vi "Dashboard Main.vi"() -> ()   [LabVIEW 2016]
uses:
  <vilib>/Utility/miscctls.llb/LVRowAndColumnTypeDef.ctl
  <vilib>/event_ctls.llb/eventvkey.ctl
  <vilib>/Rock Robotics/Network Tables/NT Read Numeric Array.vi
  <vilib>/Rock Robotics/Network Tables/NT Read Boolean.vi
  <vilib>/Rock Robotics/WPI/Dashboard/WPI_DashboardLogging Global.vi
panel:
  in  "Camera Settings Right":T1={"Frame Rate"=30, "Compression"=30, "Size"=1, "DB Camera Config"=FALSE} {"Frame Rate" scale=1.0..30.0; "Compression" scale=100.0..-1.0; "Size" items=["640x480", "320x240", "160x120"]}
  in  "Camera Name Right":string(combo)="No Camera Selection"
  out "Camera Info":cluster{"Mbps LED":bool, "Mbps":dbl, "fps":dbl} {"fps" format="%#.1g"; "Mbps" format="%#.1g"}
  in  "Camera Settings":T1={"Frame Rate"=30, "Compression"=30, "Size"=1, "DB Camera Config"=FALSE} {"Frame Rate" scale=1.0..30.0; "Compression" scale=100.0..-1.0; "Size" items=["640x480", "320x240", "160x120"]}
  in  "TCP":refnum<k5>
  in  "Rec Mode":enum32{"Stop", "Record", "Playback"}(radio)
  out "Robot IP":string
  out "Image Message":string="Timeout in Camera Communications"
  in  "Dashboard Tab":T2(tab)
  out "Centered? Cyan is go":bool
  in  "Select Auto":string(combo)="Select Autonomous ..."
  out "NT Connection":bool
  out "MotorChart R":cluster{"Numeric":dbl, "Numeric":dbl}(graph)
  out "MotorChart L":cluster{"Numeric":dbl, "Numeric":dbl}(graph)
  out "MotorSliders R":cluster{"MotorSlide1":dbl, "MotorSlide2":dbl} {"MotorSlide2" scale=-1.0..1.0 scale format="%#_2e"; "MotorSlide1" scale=-1.0..1.0 scale format="%#_2e"}
  out "MotorSliders L":cluster{"MotorSlide1":dbl, "MotorSlide2":dbl} {"MotorSlide2" scale=-1.0..1.0 scale format="%#_2e"; "MotorSlide1" scale=-1.0..1.0 scale format="%#_2e"}
  out "Gyro":dbl(knob) scale=0.0..360.0
  out "JS1 Z":dbl(slide) scale=-1.0..1.0 scale format="%#_2e"
  out "JS1 Graph":cluster{"X":dbl, "Y":dbl}[](graph)
  out "JS1 Buttons":T3
  out "JS2 Z":dbl(slide) scale=-1.0..1.0 scale format="%#_2e"
  out "JS2 Graph":cluster{"X":dbl, "Y":dbl}[](graph)
  out "JS2 Buttons":T3
  out "Mode":T4(ring)=enum."Auto Disabled"
  out "Camera Image Right":T5(plugin-control)
  in  "DB/String 9":string
  in  "DB/String 8":string
  in  "DB/String 7":string
  in  "DB/String 6":string
  in  "DB/String 5":string
  in  "DB/String 4":string
  in  "DB/String 3":string
  in  "DB/String 2":string
  in  "DB/String 1":string
  in  "DB/String 0":string
  in  "DB/Slider 0":dbl(slide) scale=0.0..5.0
  in  "DB/Slider 1":dbl(slide) scale=0.0..5.0
  in  "DB/Slider 2":dbl(slide) scale=0.0..5.0
  in  "DB/Slider 3":dbl(slide) scale=0.0..5.0
  out "DB/LED 3":bool
  out "DB/LED 2":bool
  out "DB/LED 1":bool
  out "DB/LED 0":bool
  in  "DB/Button 3":bool
  in  "DB/Button 2":bool
  in  "DB/Button 1":bool
  in  "DB/Button 0":bool caption="New Name"
  in  "Test Slider":dbl(slide) scale=0.0..100.0 scale format="%#_3g"
  in  "On/Off":bool caption="Solenoid"
  in  "Test Name":u16(ring) items=["Select the test to run..."]
  in  "Test Tree":string(tree)
  in  "Motor":cluster{"Value":dbl, "Enable":bool} {"Value" scale=-1.0..1.0 scale format="%#_3g"}
  out "Progress":T6 {"Test Progress" scale=0.0..100.0}
  in  "Rev/Fwd":cluster{"Forward":bool, "Reverse":bool}
  in  "Test Ring":u16(ring) items=["Monochrome", "Color"]
  out "Cmd Status":string
  in  "Execute Command":bool
  in  "Command Params":string[][](table)
  in  "Command Selection":i32(listbox)
  in  "CheckList":i32(listbox)
  out "Tree":string(tree)
  out "Camera Image":T5(plugin-control)
  out "Background":bool
  in  "Camera Name":string(combo)="No Camera Selection"
  # "HW"
  # "HW"
  # "Joysticks"
  # "Drive Motors"
  # "Front"
  # "Right"
  # "Left"
  # "Back"
  # "This tab is a great place for autonomous settings and robot-specific values.\nPlace controls and indicators inside this tab and match name to\nDashboard Variables on robot. You can also delete this comment."
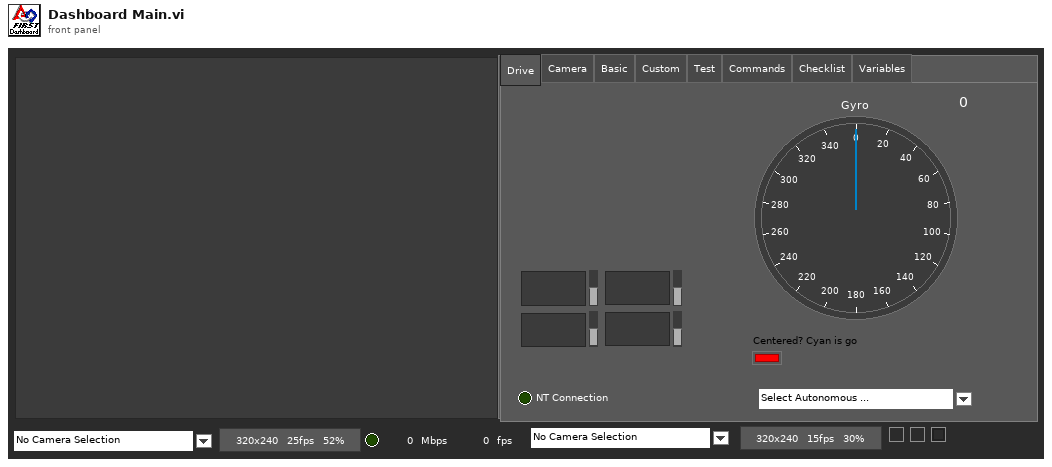
[diagram p1: front panel]
types:
  T1 = cluster{"Frame Rate":i32, "Compression":i32, "Size":u16, "DB Camera Config":bool}
  T2 = enum32{"Drive", "Camera", "Basic", "Custom", "Test", "Commands", "Checklist", "Variables"}
  T3 = cluster{bool, bool, bool, bool, bool, bool, bool, bool, bool, bool, bool, bool}
  T4 = enum8{"Tele-Op Disabled", "Tele-Op Enabled", "Auto Disabled", "Auto Enabled", "Test Disabled", "Test Enabled", "Disconnected", "No Code", "E-Stop"}
  T5 = typedef "IMAQ Image.ctl" = refnum<image>
  T6 = cluster{"Test Progress":u8, "Test Progress Text":string}
  T7 = typedef "Image Type" = u32
  T8 = cluster{"IDs":cluster{"RPC field ID":u16, "Unique ID":u16}, "String":string}
  T9 = enum32{"Drive", "Basic", "Custom", "Test", "Checklist", "Variables"}
  T10 = cluster{"Error Strings":string, "Disable Counts":cluster{u16, u16}, "Rail Faults":cluster{u16, u16, u16}, "Robot IP":string, "DB Mode":u8, "Event Info":cluster{"Name":string, "Type":u8, "Number":u16, "Replay":u8}}
  T11 = cluster{"Storage":cluster{"Disk Free":u64, "RAM Block":u32, "RAM free":u32}, "CPU Utilization":cluster{"CPU % ISR":sgl, "CPU % Time Crit":sgl, "CPU % Timed Str":sgl, "CPU % High":sgl, "CPU % Above":sgl, "CPU % Normal":sgl, "CPU % Low":sgl}, "CAN":cluster{"% Bus Utilization":sgl, "Bus Off Cnt":u32, "TX_FIFO Full Cnt":u32, "Receive Error Cnt":u8, "Transmit Error Cnt":u8}, "HID":cluster{"HID Outputs":u32, "Rumble Low":u16, "Rumble High":u16}[]}
  T12 = cluster{"Status bits":cluster{"Test Mode":bool, "Autonomous":bool, "Enabled":bool, "Code Start":bool, "Brownout":bool, "Reserved 2":bool, "Reserved 3":bool, "E-Stop":bool}, "Code Trace":cluster{"Disabled":bool, "TeleOp":bool, "Auto":bool, "Test":bool}, "Controller Type":enum16{"unknown", "cRIO", "roboRio"}, "Code?":enum16{"unknown", "noCode", "code"}, "Battery V":dbl}
  T13 = cluster{"Control Bits":cluster{"TestMode":bool, "Autonomous":bool, "Enabled":bool, "FMS Present":bool, bool, bool, bool, "E-Stop":bool}, "Team Station ":u8, "Countdown":sgl, "Joystick Values":cluster{"Axes":dbl[], "Buttons":bool[], "POVs":i16[]}[]}
  T14 = cluster{"Axes":dbl[], "Buttons":bool[], "POVs":i16[]}[]
  T15 = cluster{"Axes":dbl[], "Buttons":bool[], "POVs":i16[]}
  T16 = cluster{"Buttons[0]":bool, "Buttons[1]":bool, "Buttons[2]":bool, "Buttons[3]":bool, "Buttons[4]":bool, "Buttons[5]":bool, "Buttons[6]":bool, "Buttons[7]":bool, "Buttons[8]":bool, "Buttons[9]":bool, "Buttons[10]":bool, "Buttons[11]":bool}
  T17 = cluster{"Camera Image":refnum<vi>, "Dashboard Tab":refnum<vi>, "Background":refnum<vi>, "Rec Mode":refnum<vi>, "Test Slider":refnum<vi>, "On/Off ":refnum<vi>, "Test Ring":refnum<vi>, "Rev/Fwd":refnum<vi>, "Test Name":refnum<vi>, "Motor":refnum<vi>, "Progress":refnum<vi>, "CheckList":refnum<vi>, "Tree":refnum<vi>, "Test Tree":refnum<vi>, "Command Params":refnum<vi>, "Command Selection":refnum<vi>, "Execute Command":refnum<vi>, "Cmd Status":refnum<vi>, "Camera Settings":refnum<vi>, "Camera Name":refnum<vi>, "Camera Info":refnum<vi>, "Camera Settings Right":refnum<vi>, "Camera Name Right":refnum<vi>, "Camera Image Right":refnum<vi>}
  T18 = cluster{"Operation":enum16{"Update", "Clear"}, "Color Box":u32}[]
  T19 = typedef "eventvkey.ctl" = enum16{"ASCII", "Enter", "Return", "Shift", "Ctrl", "Alt", "Cmd", "Opt", "Caps", "NumLock", "Clear", "Break", "Up", "Down", "Left", "Right", "Insert", "Delete", "Home", "End", "PageUp", "PageDown", "Escape", "Help", "Pause", "ScrollLock", "F1", "F2", "F3", "F4", "F5", "F6", "F7", "F8", "F9", "F10", "F11", "F12", "F13", "F14", "F15", "F16", "F17", "F18", "F19", "F20", "F21", "F22", "F23", "F24", "Play", "VolumeUp", "VolumeDown", "Mute", "Two Byte Char"}
  T20 = cluster{"Image Size":bool, "Image Type":bool, "Pixel Value":bool, "ROI Information":bool, "Zoom Factor":bool}
  T21 = cluster{"Operation":enum16{"Update", "Clear"}, "Color Box":u32}
  T22 = typedef "LVRowAndColumnTypeDef.ctl" = cluster{"Row":i32, "Column":i32}
  T23 = cluster{"Shift":bool, "Ctrl":bool, "Alt":bool, "Cmd":bool, "Opt":bool}
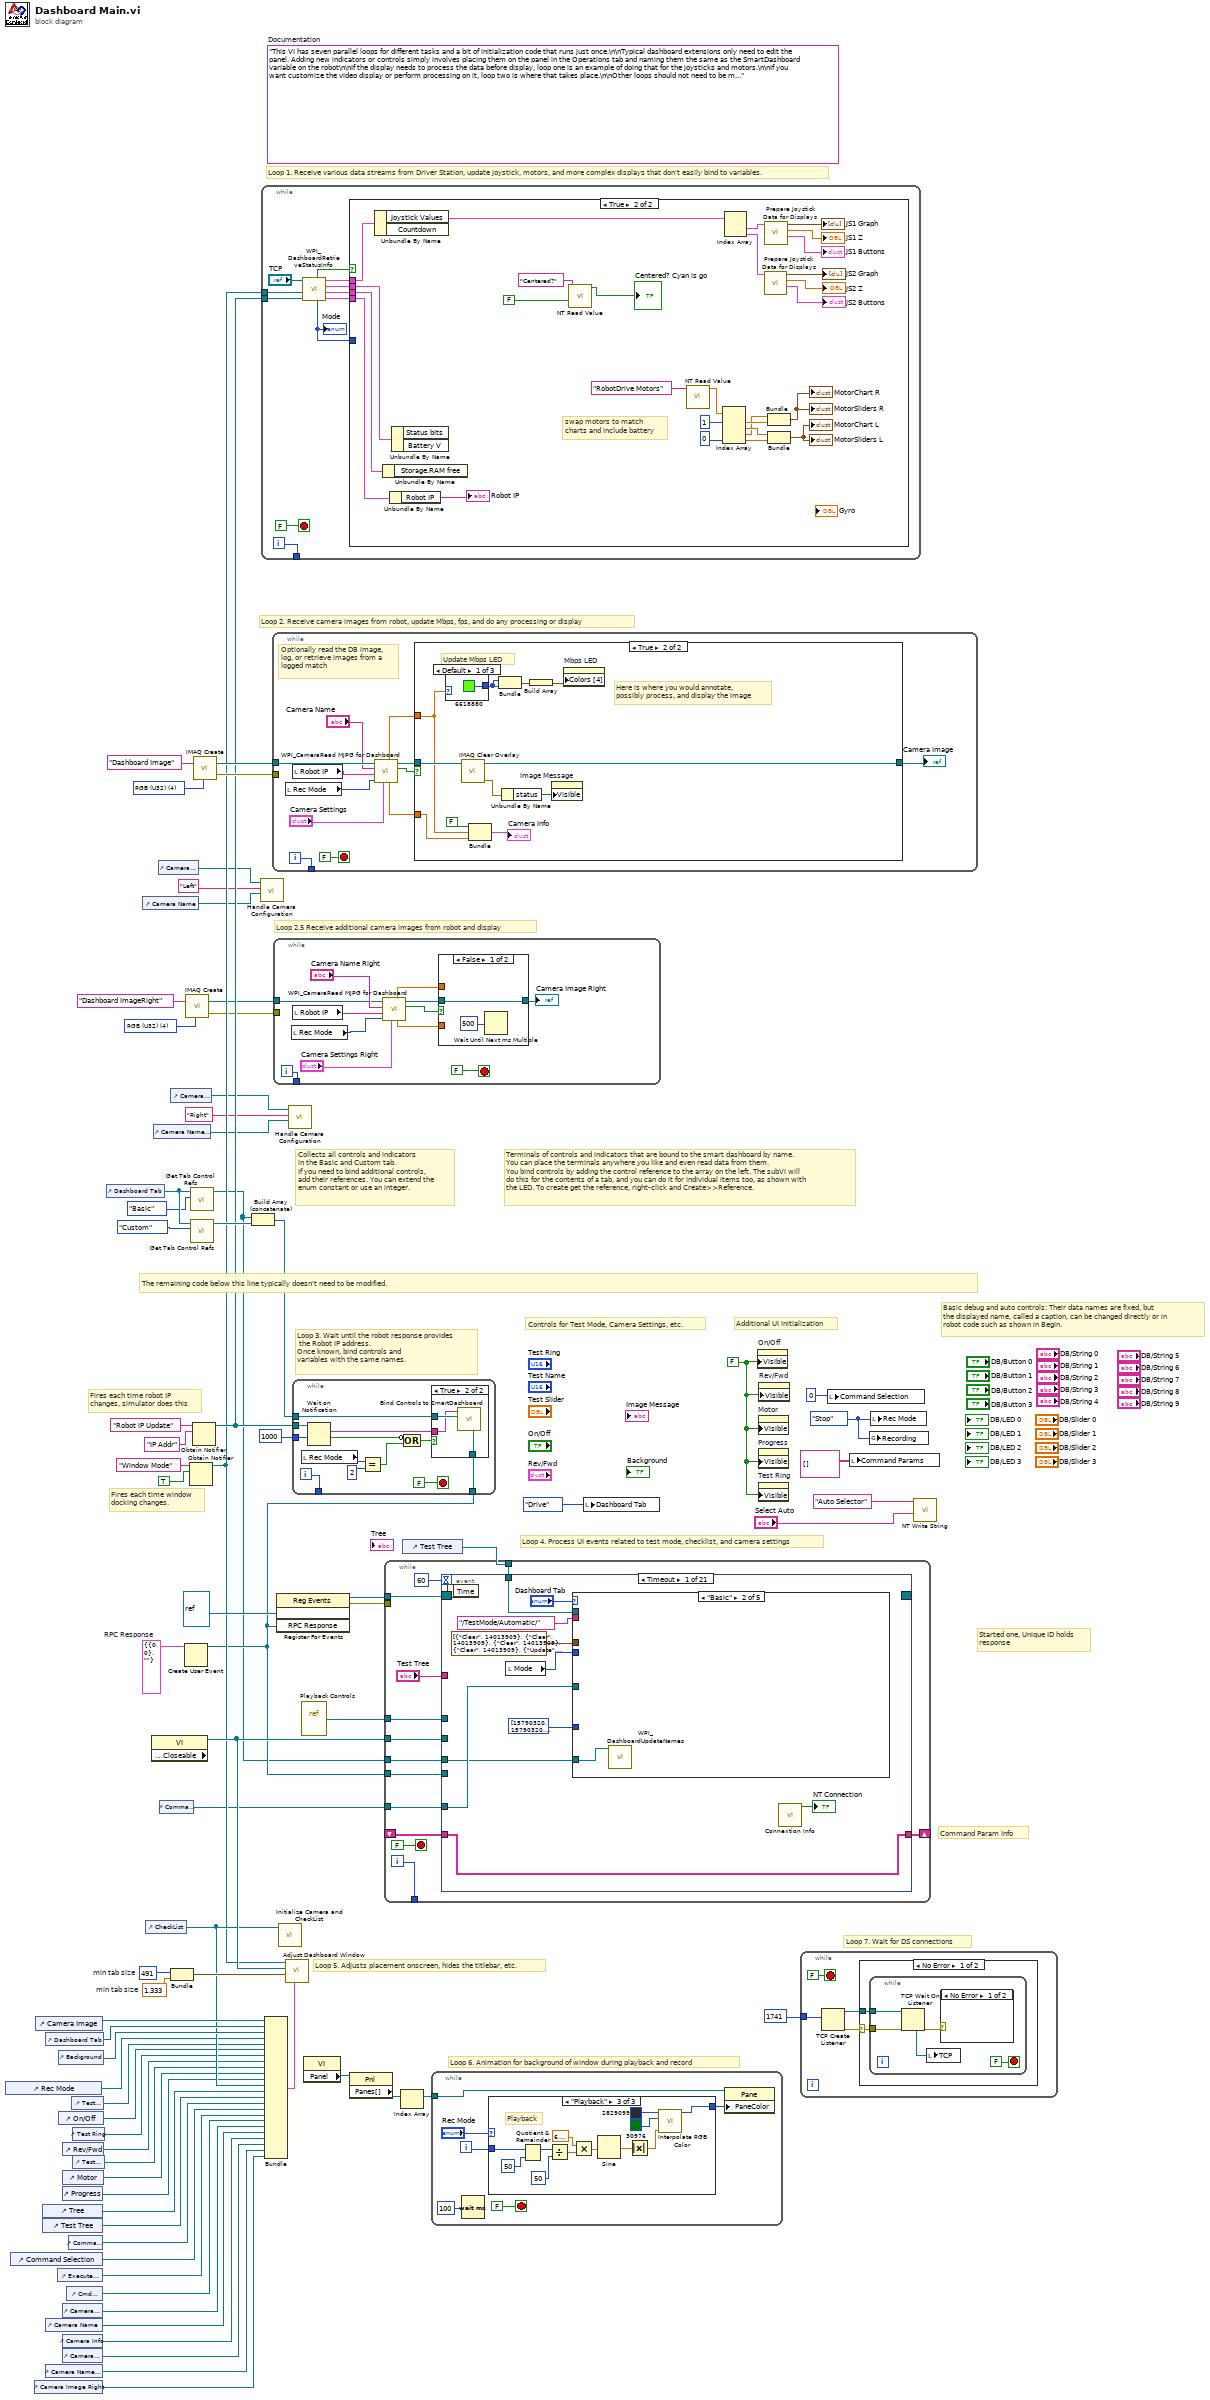
[diagram p0: block diagram]
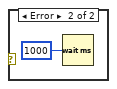
[diagram p3: hidden frame]
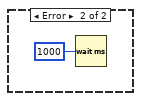
[diagram p4: hidden frame]
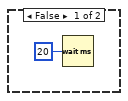
[diagram p5: hidden frame]
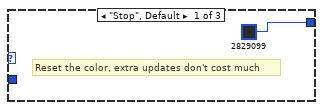
[diagram p6: hidden frame]
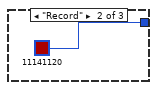
[diagram p7: hidden frame]
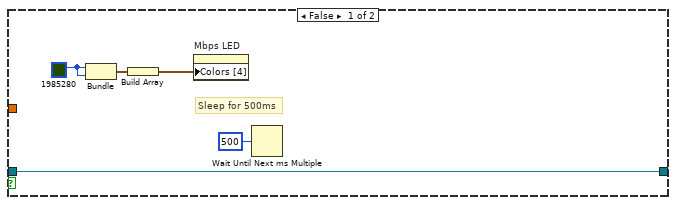
[diagram p9: hidden frame]
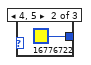
[diagram p10: hidden frame]
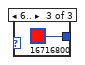
[diagram p11: hidden frame]
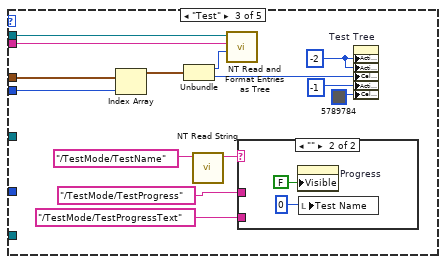
[diagram p13: hidden frame]
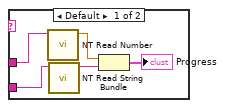
[diagram p14: hidden frame]
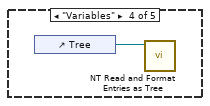
[diagram p15: hidden frame]
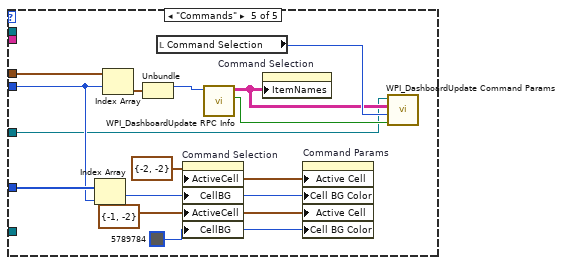
[diagram p16: hidden frame]
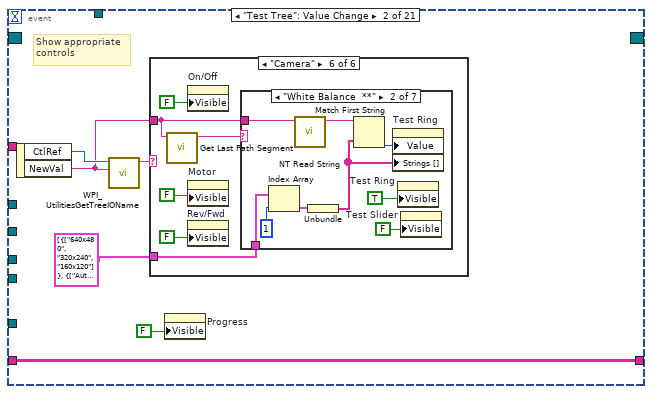
[diagram p17: hidden frame]
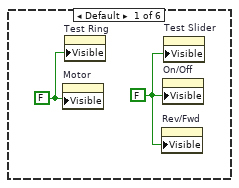
[diagram p18: hidden frame]
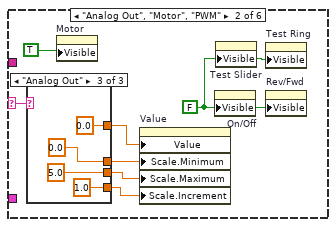
[diagram p19: hidden frame]
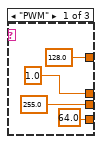
[diagram p20: hidden frame]
diagram:
  w10 = T7 4 items=["Grayscale (U8)", "Grayscale (I16)", "Grayscale (SGL)", "Complex (CSG)", "RGB (U32)", "HSL (U32)", "RGB (U64)"] ("Image Type")
  w26 = T8 {"IDs"={"RPC field ID"=0, "Unique ID"=0}, "String"=""}  # RPC Response
  w51 = 491  # min tab size
  w50 = 1.333  # min tab size
  w58 = enum32{"Stop", "Record", "Playback"}."Stop" ("Rec Mode")
  w33 = FALSE ("Visible")
  (unwired) "This VI has seven parallel loops for different tasks and a bit of initialization code that runs just once.\n\nTypical dashboard extensions only need to edit the panel. Adding new indicators or controls simply involves placing them on the panel in the Operations tab and naming them the same as the SmartDashboard variable on the robot\n\nIf the display needs to process the data before display, loop one is an example of doing that for the joysticks and motors.\n\nIf you want customize the video display or perform processing on it, loop two is where that takes place.\n\nOther loops should not need to be modified. They are pretty standard, and document the task they perform."  # Documentation
  w75 = T7 4 items=["Grayscale (U8)", "Grayscale (I16)", "Grayscale (SGL)", "Complex (CSG)", "RGB (U32)", "HSL (U32)", "RGB (U64)"] ("Image Type")
  # "Loop 2.5 Receive additional camera images from robot and display"
  # "Command Param Info"
  # "Started one, Unique ID holds\nresponse"
  # "Loop 7. Wait for DS connections"
  # "Basic debug and auto controls: Their data names are fixed, but\nthe displayed name, called a caption, can be changed directly or in\nrobot code such as shown in Begin."
  # "Controls for Test Mode, Camera Settings, etc."
  # "Additional UI Initialization"
  # "Loop 6. Animation for background of window during playback and record"
  # "Fires each time robot IP\nchanges, simulator does this"
  # "Fires each time window\ndocking changes."
  # "Collects all controls and indicators\nin the Basic and Custom tab.\nIf you need to bind additional controls,\nadd their references. You can extend the\nenum constant or use an integer."
  # "The remaining code below this line typically doesn't need to be modified."
  # "Loop 4. Process UI events related to test mode, checklist, and camera settings"
  # "Terminals of controls and indicators that are bound to the smart dashboard by name.\nYou can place the terminals anywhere you like and even read data from them.\nYou bind controls by adding the control reference to the array on the left. The subVI will\ndo this for the contents of a tab, and you can do it for individual items too, as shown with\nthe LED. To create get the reference, right-click and Create>>Reference."
  # "Loop 3. Wait until the robot response provides\n the Robot IP address.\nOnce known, bind controls and\nvariables with the same names."
  # "Loop 5. Adjusts placement onscreen, hides the titlebar, etc."
  # "Loop 1. Receive various data streams from Driver Station, update joystick, motors, and more complex displays that don't easily bind to variables."
  # "Loop 2. Receive camera images from robot, update Mbps, fps, and do any processing or display"
  n1 = control-ref of="Rec Mode"() -> (w39:refnum<vi>)
  n2 = control-ref of="Command Selection"() -> (w25:refnum<vi>)
  n3 = control-ref of="Camera Image Right"() -> (w1:refnum<vi>)
  n4 = control-ref of="Camera Image"() -> (w53:refnum<vi>)
  n5 = control-ref of="Tree"() -> (w43:refnum<vi>)
  n6 = control-ref of="Test Tree"() -> (w42:refnum<vi>)
  n7 = control-ref of="Dashboard Tab"() -> (w52:refnum<vi>)
  n8 = control-ref of="Camera Name"() -> (w16:refnum<vi>)
  n9 = control-ref of="Camera Name Right"() -> (w2:refnum<vi>)
  n10 = control-ref of="Execute Command"() -> (w27:refnum<vi>)
  n11 = control-ref of="Background"() -> (w48:refnum<vi>)
  n12 = control-ref of="On/Off"() -> (w37:refnum<vi>)
  n13 = control-ref of="Progress"() -> (w34:refnum<vi>)
  n14 = control-ref of="Camera Settings"() -> (w17:refnum<vi>)
  n15 = control-ref of="Camera Info"() -> (w15:refnum<vi>)
  n16 = control-ref of="Camera Settings Right"() -> (w3:refnum<vi>)
  n17 = control-ref of="Rev/Fwd"() -> (w35:refnum<vi>)
  n18 = control-ref of="Motor"() -> (w40:refnum<vi>)
  n19 = control-ref of="Cmd Status"() -> (w21:refnum<vi>)
  n20 = control-ref of="Command Params"() -> (w28:refnum<vi>)
  n21 = control-ref of="Test Slider"() -> (w38:refnum<vi>)
  n22 = control-ref of="Test Ring"() -> (w36:refnum<vi>)
  n23 = control-ref of="Test Name"() -> (w41:refnum<vi>)
  n24 = control-ref of="Dashboard Tab"() -> (w56:refnum<vi>)
  n25 = control-ref of="Camera Name"() -> (w18:refnum<vi>)
  n26 = control-ref of="CheckList"() -> (w44:refnum<vi>)
  n27 = property class="VI" props=["Front Panel.Closeable"]() -> (reference out=w57:refnum<vi>)  [unwired: 2 in, 2 out]
  n28 = control-ref of="Camera Name Right"() -> (w6:refnum<vi>)
  n29 = control-ref of="Camera Settings"() -> (w19:refnum<vi>)
  n30 = control-ref of="Command Params"() -> (w20:refnum<vi>)
  n31 = control-ref of="Camera Settings Right"() -> (w7:refnum<vi>)
  n32 = Bundle("min tab size"=w51, "min tab size"=w50) -> (w49:cluster{"min tab size":i32, "min tab size":dbl})  [unwired: 1 in]
  n33 = Create User Event(user event datatype=w26) -> (user event=w22:refnum<user-event>)  [unwired: 1 in, 1 out]
  n34 = call "IMAQ Create"("Image Name"="Dashboard ImageRight", "Image Type"=w10) -> ("New Image"=w9:T5, "error out"=w8:errorcluster)  [unwired: 2 in, 1 out]
  n35 = Obtain Notifier(name (unnamed)="Window Mode", notification data type=TRUE) -> (notifier out=w31:refnum<notifier>)  [unwired: 2 in, 2 out]
  n36 = call <vilib>:"Get Tab Control Refs.vi"("Page Index"=T9."Basic" ("Dashboard Tab"), "TabControl in"=w56) -> ("ControlsOnPage"=w14:refnum<vi>[])  [unwired: 9 in]
  n37 = call <vilib>:"Get Tab Control Refs.vi"("Page Index"=T9."Custom" ("Dashboard Tab"), "TabControl in"=w56) -> ("ControlsOnPage"=w55:refnum<vi>[])  [unwired: 9 in]
  n38 = Obtain Notifier(name (unnamed)="Robot IP Update", notification data type="IP Addr" ("name (unnamed)")) -> (notifier out=w32:refnum<notifier>)  [unwired: 2 in, 2 out]
  n39 = call "IMAQ Create"("Image Name"="Dashboard Image", "Image Type"=w75) -> ("New Image"=w73:T5, "error out"=w72:errorcluster)  [unwired: 2 in, 1 out]
  n40 = Build Array (concatenate)(w14, w55) -> (w54:refnum<vi>[])
  n41 = call "Handle Camera Configuration.vi"("CameraNameRef"=w18, "Camera File Name"="Left", "ClusterRef"=w19) -> ()  [unwired: 9 in]
  n42 = while {
    tunnel: [w85] -> _
    tunnel: w32 -> [w79]
    tunnel: w31 -> [w76]
    i -> [w85]
    stop <- FALSE stop-if-true
    n43 = call <vilib>:"WPI_DashboardRetrieveStatusInfo.vi"("Binding Refnum"=w79, "Window Mode Notifier"=w76, "TCP Cnx"="TCP") -> ("Power and Errors"=w80:T10, "Robot Metrics"=w83:T11, "Status Info"=w84:T12, "Control Info"=w81:T13, "Robot Mode"=w78:T4, "Process?"=w82:bool)  [unwired: 3 in]
    "Mode" <- w78
    n44 = case shown="True" w82 {
      tunnel: w84 -> [_ w114]
      tunnel: w83 -> [_ w113]
      tunnel: w81 -> [_ w112]
      tunnel: w80 -> [_ w111]
      tunnel: w78 -> [_ _]
      frame False {
        n45 = Wait (ms)(milliseconds to wait=u32 20) -> ()  [unwired: 1 out]
      }
      frame True {
        # "swap motors to match\ncharts and include battery"
        n46 = Unbundle By Name(w112) -> ("Joystick Values"=w102:T14)  [unwired: 1 out]
        n47 = Unbundle By Name(w113) -> ()  [unwired: 1 out]
        n48 = Unbundle By Name(w111) -> ("Robot IP"=→"Robot IP":string)
        n49 = Unbundle By Name(w114) -> ()  [unwired: 2 out]
        n50 = call-poly <vilib>:"NT Read Value.vi"("Default Value"=FALSE, "Name"="Centered?") -> ("Boolean"=→"Centered? Cyan is go":bool)  [unwired: 8 in, 1 out]
        n51 = call-poly <vilib>:"NT Read Value.vi"("Name"="RobotDrive Motors") -> ("Numeric Array"=w92:dbl[])  [unwired: 9 in, 1 out]
        n52 = Index Array(array=w92, index #1=1, index #4=0) -> (element #1=w106:dbl, element #2=w107:dbl, element #3=w105:dbl, element #4=w110:dbl)  [unwired: 2 in]
        n53 = Index Array(array=w102) -> (element #1=w101:T15, element #2=w97:T15)  [unwired: 2 in]
        n54 = call "Prepare Joystick Data for Displays.vi"("Joystick Values"=w97) -> ("Buttons"=→"JS2 Buttons":T16, "Z Axis"=→"JS2 Z":dbl, "Cartesian Data"=→"JS2 Graph":cluster{"X axis":dbl, "X axis":dbl}[])  [unwired: 8 in]
        n55 = call "Prepare Joystick Data for Displays.vi"("Joystick Values"=w101) -> ("Buttons"=→"JS1 Buttons":T16, "Z Axis"=→"JS1 Z":dbl, "Cartesian Data"=→"JS1 Graph":cluster{"X axis":dbl, "X axis":dbl}[])  [unwired: 8 in]
        n56 = Bundle("Numeric"=w105, "Numeric"=w106) -> (→"MotorChart R" →"MotorSliders R":cluster{"Numeric":dbl, "Numeric":dbl})  [unwired: 1 in]
        n57 = Bundle("Numeric"=w107, "Numeric"=w110) -> (→"MotorChart L" →"MotorSliders L":cluster{"Numeric":dbl, "Numeric":dbl})  [unwired: 1 in]
      }
    }
  }
  n58 = Bundle("Camera Image"=w53, "Dashboard Tab"=w52, "Background"=w48, "Rec Mode"=w39, "Test Slider"=w38, "On/Off"=w37, "Test Ring"=w36, "Rev/Fwd"=w35, "Test Name"=w41, "Motor"=w40, "Progress"=w34, "CheckList"=w44, "Tree"=w43, "Test Tree"=w42, "Command Params"=w28, "Command Selection"=w25, "Execute Command"=w27, "Cmd Status"=w21, "Camera Settings"=w17, "Camera Name"=w16, "Camera Info"=w15, "Camera Settings Right"=w3, "Camera Name Right"=w2, "Camera Image Right"=w1) -> (w45:T17)  [unwired: 1 in]
  n59 = while {
    tunnel: w73 -> [w124]
    tunnel: w72 -> [_]
    tunnel: [w125] -> _
    i -> [w125]
    stop <- FALSE stop-if-true
    # "Optionally read the DB image,\nlog, or retrieve images from a\nlogged match"
    n60 = local read "Rec Mode"() -> (w120:enum32{"Stop", "Record", "Playback"})
    n61 = local read "Robot IP"() -> (w119:string)
    n62 = call <vilib>:"WPI_CameraRead MJPG for Dashboard.vi"("Camera Settings"="Camera Settings", "Rec Mode"=w120, "Robot IP"=w119, "Camera Name"="Camera Name", "Refnum in"=w124) -> ("Active"=w122:bool, "Refnum out"=w123:T5, "FPS"=w121:dbl, "Bandwidth (Mbps)"=w118:dbl)  [unwired: 3 in]
    n63 = case shown="True" w122 {
      tunnel: w123 -> [w127 w138]
      tunnel: w118 -> [_ w135]
      tunnel: w121 -> [_ w136]
      tunnel: [w127 w132] -> w115
      frame False {
        w129 = u32 1985280 ("Color Box")
        # "Sleep for 500ms"
        n64 = Bundle("Color Box"=w129, "Color Box"=w129) -> (w130:cluster{"Color Box":u32, "Color Box":u32})  [unwired: 1 out]
        n65 = Build Array(w130) -> (w128:cluster{"Color Box":u32, "Color Box":u32}[])
        n66 = property on="Mbps LED" class="Bool (strict)"("Colors [4]"=w128) -> ()  [unwired: 2 in, 2 out]
        n67 = Wait Until Next ms Multiple(millisecond multiple=u32 500) -> ()  [unwired: 1 out]
      }
      frame True {
        # "Here is where you would annotate,\npossibly process, and display the image"
        # "Update Mbps LED"
        n68 = case shown="Default" w135 {
          tunnel: [u32 6618880 ("Color Box") u32 16776722 ("Color Box") u32 16716800 ("Color Box")] -> w139
          frame Default {
          }
          frame 4, 5 {
          }
          frame 6.. {
          }
        }
        n69 = call "IMAQ Clear Overlay"("Image"=w138) -> ("error out"=w141:errorcluster, "Image Out"=w132:T5)  [unwired: 2 in, 7 out]
        n70 = Bundle(FALSE, "Bandwidth (Mbps)"=w135, "FPS"=w136) -> (→"Camera Info":cluster{bool, "Bandwidth (Mbps)":dbl, "FPS":dbl})  [unwired: 1 in]
        n71 = Bundle("Color Box"=w139, "Color Box"=w139) -> (w140:cluster{"Color Box":u32, "Color Box":u32})  [unwired: 1 out]
        n72 = Unbundle By Name(w141) -> ("status"=w142:bool)
        n73 = Build Array(w140) -> (w137:cluster{"Color Box":u32, "Color Box":u32}[])
        n74 = property on="Image Message" class="Str"("Visible"=w142) -> ()  [unwired: 2 in, 2 out]
        n75 = property on="Mbps LED" class="Bool (strict)"("Colors [4]"=w137) -> ()  [unwired: 2 in, 2 out]
      }
    }
    "Camera Image" <- w115
  }
  n76 = while {
    tunnel: w9 -> [w156]
    tunnel: w8 -> [_]
    tunnel: [w150] -> _
    i -> [w150]
    stop <- FALSE stop-if-true
    n77 = local read "Rec Mode"() -> (w154:enum32{"Stop", "Record", "Playback"})
    n78 = local read "Robot IP"() -> (w155:string)
    n79 = call <vilib>:"WPI_CameraRead MJPG for Dashboard.vi"("Camera Settings"="Camera Settings Right", "Rec Mode"=w154, "Robot IP"=w155, "Camera Name"="Camera Name Right", "Refnum in"=w156) -> ("Active"=w149:bool, "Refnum out"=w152:T5, "FPS"=w147:dbl, "Bandwidth (Mbps)"=w148:dbl)  [unwired: 3 in]
    n80 = case shown="False" w149 {
      tunnel: w152 -> [w158 w160]
      tunnel: w148 -> [_ _]
      tunnel: w147 -> [_ _]
      tunnel: [w158 w160] -> w146
      frame False {
        n81 = Wait Until Next ms Multiple(millisecond multiple=u32 500) -> ()  [unwired: 1 out]
      }
      frame True {
      }
    }
    "Camera Image Right" <- w146
  }
  n82 = register-events(refnum<vi> refnum, w22) -> (reference out=w62:refnum<event-registration>, error out=w61:errorcluster)  [unwired: 2 in]
  n83 = call "Initialize Camera and CheckList.vi"("ListBox in"=w44) -> ()  [unwired: 11 in]
  n84 = call "Adjust Dashboard Window.vi"("Sizing Refnums"=w45, "Size Constraints"=w49, "VI"=w57, "WIn Mode"=w31) -> ()  [unwired: 8 in]
  n85 = call "Handle Camera Configuration.vi"("CameraNameRef"=w6, "Camera File Name"="Right", "ClusterRef"=w7) -> ()  [unwired: 9 in]
  n86 = while {
    tunnel: w54 -> [w172]
    tunnel: w32 -> [w170]
    tunnel: [w168] -> _
    tunnel: u32 1000 ("milliseconds to wait") -> [w167]
    tunnel: w22 -> [w161]
    i -> [w168]
    stop <- FALSE stop-if-true
    n87 = local read "Rec Mode"() -> (w163:enum32{"Stop", "Record", "Playback"})
    n88 = Wait on Notification(notifier=w170, timeout in ms (-1)=w167) -> (notification=w169:string, timed out?=w165:bool)  [unwired: 2 in, 2 out]
    n89 = Equal?(x=w163, y=u16 2 ("Rec Mode")) -> (x = y?=w164:bool)
    n90 = Compound Arithmetic op=OR(invert w165, w164) -> (w166:bool)
    n91 = case shown="True" w166 {
      tunnel: w172 -> [_ w175]
      tunnel: w169 -> [_ w174]
      tunnel: w161 -> [_ w173]
      frame False {
      }
      frame True {
        n92 = call <vilib>:"Bind Controls to SmartDashboard.vi"("RPC ref"=w173, "Bound Control Refs"=w175, "Server IP Address"=w174) -> ()  [unwired: 9 in]
      }
    }
  }
  n93 = vi-ref "Playback Controls.vi"() -> (w63:refnum<vi>)
  n94 = property class="VI"() -> ("Panel"=w65:refnum<vi>)  [unwired: 2 in, 2 out]
  n95 = property class="Pnl"(reference=w65) -> ("Panes[]"=w66:refnum<vi>[])  [unwired: 1 in, 2 out]
  n96 = Index Array(array=w66) -> (element=w64:refnum<vi>)  [unwired: 1 in]
  n97 = control-ref of="Test Tree"() -> (w67:refnum<vi>)
  n98 = while {
    tunnel: [w185] -> _
    tunnel: w67 -> [w184]
    tunnel: w63 -> [w183]
    tunnel: w62 -> [w182]
    tunnel: w61 -> [_]
    tunnel: w57 -> [w181]
    tunnel: w22 -> [w180]
    tunnel: w20 -> [w179]
    shift-right: [w178] -> _
    shift-left: _ -> [w177]
    tunnel: w14 -> [w176]
    i -> [w185]
    stop <- FALSE stop-if-true
    n99 = event shown="[0] Timeout" {
      selector: w182 -> [_ _ _ _ _ _ _ _ _ _ _ _ _ _ _ _ _ _ _ _ _]
      dyn-events: [_ _ _ _ _ _ _ _ _ _ _ _ _ _ _ _ w441 _ _ _ _] -> _
      timeout: u32 60 ("milliseconds to wait") -> [_ _ _ _ _ _ _ _ _ _ _ _ _ _ _ _ _ _ _ _ _]
      tunnel: w184 -> [w197 _ _ _ _ _ _ _ _ _ _ _ _ _ _ _ _ _ _ _ _]
      tunnel: "Test Tree" -> [_ _ _ _ _ _ _ _ _ _ _ w408 w416 w418 w422 w430 _ _ _ _ _]
      tunnel: w183 -> [_ _ _ _ _ _ _ _ _ _ _ _ _ _ _ _ w443 _ w461 _ _]
      tunnel: w181 -> [_ _ _ _ _ _ _ _ _ _ _ _ _ _ _ _ w439 _ _ _ _]
      tunnel: w180 -> [_ _ _ _ _ _ _ _ _ _ _ _ _ _ _ _ w435 _ _ _ _]
      tunnel: w179 -> [w192 _ _ _ _ _ w359 _ _ _ _ _ _ _ _ _ _ _ _ _ _]
      tunnel: [w191 w236 w338 w343 w352 w356 w357 w366 w376 w383 w395 w407 w414 w417 w421 w429 w434 w456 w458 w462 w473] -> w178
      tunnel: w177 -> [w191 w236 w338 w343 w352 w356 w357 _ _ w383 w395 w407 w414 w417 w421 w429 w434 w456 w458 w462 w473]
      tunnel: w176 -> [w189 _ _ _ _ _ _ _ _ _ _ _ _ _ _ _ _ _ _ _ _]
      event Timeout {
        n100 = event-data() -> ()  [unwired: 1 in, 1 out]
        n101 = local read "Mode"() -> (w194:T4)
        n102 = case shown="\"Basic\"" "Dashboard Tab" {
          tunnel: w197 -> [_ _ w213 _ _]
          tunnel: "/TestMode/Automatic/" ("Name Pattern") -> [_ _ w212 _ _]
          tunnel: T18 [{"Operation"=enum."Clear", "Color Box"=14013909}, {"Operation"=enum."Clear", "Color Box"=14013909}, {"Operation"=enum."Clear", "Color Box"=14013909}, {"Operation"=enum."Clear", "Color Box"=14013909}, {"Operation"=enum."Update", "Color Box"=14013909}, {"Operation"=enum."Update", "Color Box"=16777215}, {"Operation"=enum."Clear", "Color Box"=14013909}, {"Operation"=enum."Clear", "Color Box"=14013909}, {"Operation"=enum."Clear", "Color Box"=14013909}] -> [_ _ w205 _ w229]
          tunnel: w194 -> [_ _ w204 _ w228]
          tunnel: u32[] [15790320, 15790320, 15790320, 15790320, 16777215, 16777215, 15790320, 15790320, 15790320] -> [_ _ _ _ w234]
          tunnel: w192 -> [_ _ _ _ w222]
          tunnel: w189 -> [_ w199 _ _ _]
          frame "Custom", Default {
          }
          frame "Basic" {
            n103 = call <vilib>:"WPI_DashboardUpdateNames.vi"("Controls on Tab"=w199) -> ()  [unwired: 11 in]
          }
          frame "Test" {
            w211 = -2 ("Active Item:Row Number")
            n104 = Index Array(array=w205, index=w204) -> (element=w206:T21)
            n105 = Unbundle(w206) -> ("Operation"=w207:enum16{"Update", "Clear"}, "Color Box"=w208:u32)
            n106 = call <vilib>:"NT Read String.vi"("Name"="/TestMode/TestName") -> ("String"=w202:string)  [unwired: 9 in, 1 out]
            n107 = call <vilib>:"NT Read and Format Entries as Tree.vi"("Operation"=w207, "Name Pattern"=w212, "Tree Refnum"=w213) -> ()  [unwired: 7 in, 2 out]
            n108 = case shown="\"\"" w202 {
              tunnel: "/TestMode/TestProgress" ("Name") -> [w215 _]
              tunnel: "/TestMode/TestProgressText" ("Name") -> [w214 _]
              frame Default {
                n109 = call <vilib>:"NT Read Number.vi"("Name"=w215) -> ("Numeric"=w216:dbl)  [unwired: 9 in, 1 out]
                n110 = call <vilib>:"NT Read String.vi"("Name"=w214) -> ("String"=w217:string)  [unwired: 9 in, 1 out]
                n111 = Bundle("Numeric"=w216, "String"=w217) -> (→"Progress":cluster{"Numeric":dbl, "String":string})  [unwired: 1 in]
              }
              frame "" {
                n112 = property on="Progress" class="Clust (strict)"("Visible"=FALSE) -> ()  [unwired: 2 in, 2 out]
                n113 = local write "Test Name"(u16 0) -> ()
              }
            }
            n114 = property on="Test Tree" class="Tree (strict)"("Active Item Row Number"=w211, "ActiveColNum"=w211, "CellBG"=w208, "Active Item Row Number"=-1 ("Active Item:Row Number"), "CellBG"=u32 5789784 ("Color Box")) -> ()  [unwired: 2 in, 2 out]
          }
          frame "Variables" {
            n115 = control-ref of="Tree"() -> (w221:refnum<vi>)
            n116 = call <vilib>:"NT Read and Format Entries as Tree.vi"("Tree Refnum"=w221) -> ()  [unwired: 9 in, 2 out]
          }
          frame "Commands" {
            w230 = u32 5789784 ("Color Box")
            w231 = T22 {"Row"=-1, "Column"=-2} ("Active Cell:Active Cell")
            w233 = T22 {"Row"=-2, "Column"=-2} ("Active Cell:Active Cell")
            n117 = Index Array(array=w234, index=w228) -> (element=w232:u32)
            n118 = Index Array(array=w229, index=w228) -> (element=w227:T21)
            n119 = Unbundle(w227) -> ("Operation"=w226:enum16{"Update", "Clear"})  [unwired: 1 out]
            n120 = local read "Command Selection"() -> (w225:i32)
            n121 = property on="Command Selection" class="MCListbox (strict)"("ActiveCell"=w233, "CellBG"=w232, "ActiveCell"=w231, "CellBG"=w230) -> ()  [unwired: 2 in, 2 out]
            n122 = call <vilib>:"WPI_DashboardUpdate RPC Info.vi"("Operation"=w226) -> ("update"=w224:bool, "commands"=w223:string[][])  [unwired: 9 in]
            n123 = property on="Command Selection" class="MCListbox (strict)"("ItemNames"=w223) -> ()  [unwired: 2 in, 2 out]
            n124 = property on="Command Params" class="Tbl (strict)"("Active Cell"=w233, "Cell BG Color"=w232, "Active Cell"=w231, "Cell BG Color"=w230) -> ()  [unwired: 2 in, 2 out]
            n125 = call <vilib>:"WPI_DashboardUpdate Command Params.vi"("Update"=w224, "NewVal"=w225, "Commands"=w223, "Param Tbl"=w222) -> ()  [unwired: 7 in, 1 out]
          }
        }
        n126 = call <vilib>:"Connextion Info.vi"() -> ("Connected"=→"NT Connection":bool)  [unwired: 10 in, 1 out]
      }
      event "Test Tree": Value Change {
        # "Show appropriate\ncontrols"
        n127 = event-data() -> ("CtlRef"=w239:refnum<vi>, "NewVal"=w237:string)  [unwired: 1 in]
        n128 = call <vilib>:"WPI_UtilitiesGetTreeIOName.vi"("NewVal"=w237, "TreeControl in"=w239) -> ("I/O Name"=w240:string)  [unwired: 9 in]
        n129 = case shown="\"Camera\"" w240 {
          selector: w240 -> [_ w247 _ w269 w278 _]
          tunnel: w237 -> [_ _ w266 w268 _ w285]
          tunnel: cluster{string[]}[] [{["640x480", "320x240", "160x120"]}, {["Auto", "Fixed indoor", "Fixed outdoor 1", "Fixed outdoor 2", "Fixed fluorescent 1", "Fixed fluorescent 2", "Hold current"]}, {["Auto", "Flicker-free 50 Hz", "Flicker-free 60 Hz", "Hold current"]}, {["None", "Prioritize frame rate", "Prioritize image quality"]}, {["Monochrome", "Color"]}] -> [_ _ _ _ _ w284]
          frame Default {
            w242 = FALSE ("Visible")
            w241 = FALSE ("Visible")
            n130 = property on="Motor" class="Clust (strict)"("Visible"=w241) -> ()  [unwired: 2 in, 2 out]
            n131 = property on="Test Ring" class="Ring (strict)"("Visible"=w241) -> ()  [unwired: 2 in, 2 out]
            n132 = property on="Rev/Fwd" class="Clust (strict)"("Visible"=w242) -> ()  [unwired: 2 in, 2 out]
            n133 = property on="On/Off" class="Bool (strict)"("Visible"=w242) -> ()  [unwired: 2 in, 2 out]
            n134 = property on="Test Slider" class="Slide (strict)"("Visible"=w242) -> ()  [unwired: 2 in, 2 out]
          }
          frame "Analog Out", "Motor", "PWM" {
            w248 = FALSE ("Visible")
            n135 = case shown="\"Analog Out\"" w247 {
              tunnel: [1.0 ("Value") -1.0 ("Value") 0.0 ("Value")] -> w246
              tunnel: [255.0 ("Value") 1.0 ("Value") 5.0 ("Value")] -> w245
              tunnel: [128.0 ("Value") 0.0 ("Value") 0.0 ("Value")] -> w244
              tunnel: [64.0 ("Value") 0.5 ("Value") 1.0 ("Value")] -> w243
              frame "PWM" {
              }
              frame "Motor", Default {
              }
              frame "Analog Out" {
              }
            }
            n136 = property on="Motor" class="Clust (strict)"("Visible"=TRUE) -> ()  [unwired: 2 in, 2 out]
            n137 = property on="Value" class="Slide (strict)"("Value"=w244, "Scale.Minimum"=w246, "Scale.Maximum"=w245, "Scale.Increment"=w243) -> ()  [unwired: 2 in, 2 out]
            n138 = property on="On/Off" class="Bool (strict)"("Visible"=w248) -> ()  [unwired: 2 in, 2 out]
            n139 = property on="Test Slider" class="Slide (strict)"("Visible"=w248) -> ()  [unwired: 2 in, 2 out]
            n140 = property on="Test Ring" class="Ring (strict)"("Visible"=w248) -> ()  [unwired: 2 in, 2 out]
            n141 = property on="Rev/Fwd" class="Clust (strict)"("Visible"=w248) -> ()  [unwired: 2 in, 2 out]
          }
          frame "Servo" {
            w264 = FALSE ("Visible")
            n142 = call <vilib>:"NT Read Number.vi"("Name"=w266) -> ("Numeric"=w265:dbl)  [unwired: 9 in, 1 out]
            n143 = property on="Test Slider" class="Slide (strict)"("Visible"=TRUE, "Scale.Maximum"=170.0 ("Scale.Range:Maximum")) -> ()  [unwired: 2 in, 2 out]
            n144 = local write "Test Slider"(w265) -> ()
            n145 = property on="Motor" class="Clust (strict)"("Visible"=w264) -> ()  [unwired: 2 in, 2 out]
            n146 = property on="Rev/Fwd" class="Clust (strict)"("Visible"=w264) -> ()  [unwired: 2 in, 2 out]
            n147 = property on="On/Off" class="Bool (strict)"("Visible"=w264) -> ()  [unwired: 2 in, 2 out]
            n148 = property on="Test Ring" class="Ring (strict)"("Visible"=w264) -> ()  [unwired: 2 in, 2 out]
          }
          frame "Relay", "Solenoid" {
            w267 = FALSE ("Visible")
            n149 = property on="Motor" class="Clust (strict)"("Visible"=w267) -> ()  [unwired: 2 in, 2 out]
            n150 = property on="Test Slider" class="Slide (strict)"("Visible"=w267) -> ()  [unwired: 2 in, 2 out]
            n151 = Search and Replace String(input string=w268, search string="/Value  **", replace string="/Direction") -> (result string=w274:string)  [unwired: 5 in, 3 out]
            n152 = property on="Test Ring" class="Ring (strict)"("Visible"=w267) -> ()  [unwired: 2 in, 2 out]
            n153 = call <vilib>:"NT Read String.vi"("Name"=w274) -> ("String"=w272:string)  [unwired: 9 in, 1 out]
            n154 = Equal?(x="Both directions", y=w272) -> (x = y?=w270:bool)
            n155 = Not(x=w270) -> (.not. x?=w271:bool)
            n156 = property on="Rev/Fwd" class="Clust (strict)"("Visible"=w270) -> ()  [unwired: 2 in, 2 out]
            n157 = property on="On/Off" class="Bool (strict)"("Visible"=w271, "Caption.Text"=w269) -> ()  [unwired: 2 in, 2 out]
          }
          frame "Compressor", "Digital Out" {
            w277 = FALSE ("Visible")
            # "Get direction and finish"
            n158 = property on="Motor" class="Clust (strict)"("Visible"=w277) -> ()  [unwired: 2 in, 2 out]
            n159 = property on="Test Slider" class="Slide (strict)"("Visible"=w277) -> ()  [unwired: 2 in, 2 out]
            n160 = property on="Test Ring" class="Ring (strict)"("Visible"=w277) -> ()  [unwired: 2 in, 2 out]
            n161 = property on="On/Off" class="Bool (strict)"("Visible"=TRUE, "Caption.Text"=w278) -> ()  [unwired: 2 in, 2 out]
            n162 = property on="Rev/Fwd" class="Clust (strict)"("Visible"=FALSE) -> ()  [unwired: 2 in, 2 out]
          }
          frame "Camera" {
            n163 = call <vilib>:"Get Last Path Segment.vi"("String in"=w285) -> ("String out"=w286:string)  [unwired: 10 in]
            n164 = property on="On/Off" class="Bool (strict)"("Visible"=FALSE) -> ()  [unwired: 2 in, 2 out]
            n165 = property on="Motor" class="Clust (strict)"("Visible"=FALSE) -> ()  [unwired: 2 in, 2 out]
            n166 = property on="Rev/Fwd" class="Clust (strict)"("Visible"=FALSE) -> ()  [unwired: 2 in, 2 out]
            n167 = case shown="\"White Balance  **\"" w286 {
              tunnel: w285 -> [w292 w301 w310 w319 w328 _ w334]
              tunnel: w284 -> [w290 w298 w307 w316 w325 _ _]
              frame "Size  **" {
                n168 = Index Array(array=w290) -> (element=w289:cluster{string[]})  [unwired: 1 in]
                n169 = call <vilib>:"NT Read String.vi"("Name"=w292) -> ("String"=w291:string)  [unwired: 9 in, 1 out]
                n170 = Unbundle(w289) -> (w287:string[])
                n171 = Match First String(2:w287, 3:w291) -> (0:w288:i32)  [unwired: 1 out]
                n172 = property on="Test Ring" class="Ring (strict)"("Value"=w288, "Strings []"=w287) -> ()  [unwired: 2 in, 2 out]
                n173 = property on="Test Ring" class="Ring (strict)"("Visible"=TRUE) -> ()  [unwired: 2 in, 2 out]
                n174 = property on="Test Slider" class="Slide (strict)"("Visible"=FALSE) -> ()  [unwired: 2 in, 2 out]
              }
              frame "White Balance  **" {
                n175 = Index Array(array=w298, index=1) -> (element=w299:cluster{string[]})
                n176 = call <vilib>:"NT Read String.vi"("Name"=w301) -> ("String"=w300:string)  [unwired: 9 in, 1 out]
                n177 = Unbundle(w299) -> (w296:string[])
                n178 = Match First String(2:w296, 3:w300) -> (0:w295:i32)  [unwired: 1 out]
                n179 = property on="Test Ring" class="Ring (strict)"("Value"=w295, "Strings []"=w296) -> ()  [unwired: 2 in, 2 out]
                n180 = property on="Test Ring" class="Ring (strict)"("Visible"=TRUE) -> ()  [unwired: 2 in, 2 out]
                n181 = property on="Test Slider" class="Slide (strict)"("Visible"=FALSE) -> ()  [unwired: 2 in, 2 out]
              }
              frame "Exposure  **" {
                n182 = Index Array(array=w307, index=2) -> (element=w308:cluster{string[]})
                n183 = call <vilib>:"NT Read String.vi"("Name"=w310) -> ("String"=w309:string)  [unwired: 9 in, 1 out]
                n184 = Unbundle(w308) -> (w304:string[])
                n185 = Match First String(2:w304, 3:w309) -> (0:w305:i32)  [unwired: 1 out]
                n186 = property on="Test Ring" class="Ring (strict)"("Value"=w305, "Strings []"=w304) -> ()  [unwired: 2 in, 2 out]
                n187 = property on="Test Ring" class="Ring (strict)"("Visible"=TRUE) -> ()  [unwired: 2 in, 2 out]
                n188 = property on="Test Slider" class="Slide (strict)"("Visible"=FALSE) -> ()  [unwired: 2 in, 2 out]
              }
              frame "Exposure Priority  **" {
                n189 = Index Array(array=w316, index=3) -> (element=w317:cluster{string[]})
                n190 = call <vilib>:"NT Read String.vi"("Name"=w319) -> ("String"=w318:string)  [unwired: 9 in, 1 out]
                n191 = Unbundle(w317) -> (w313:string[])
                n192 = Match First String(2:w313, 3:w318) -> (0:w314:i32)  [unwired: 1 out]
                n193 = property on="Test Ring" class="Ring (strict)"("Value"=w314, "Strings []"=w313) -> ()  [unwired: 2 in, 2 out]
                n194 = property on="Test Ring" class="Ring (strict)"("Visible"=TRUE) -> ()  [unwired: 2 in, 2 out]
                n195 = property on="Test Slider" class="Slide (strict)"("Visible"=FALSE) -> ()  [unwired: 2 in, 2 out]
              }
              frame "Color Enable  **" {
                n196 = Index Array(array=w325, index=4) -> (element=w326:cluster{string[]})
                n197 = call <vilib>:"NT Read String.vi"("Name"=w328) -> ("String"=w327:string)  [unwired: 9 in, 1 out]
                n198 = Unbundle(w326) -> (w322:string[])
                n199 = Match First String(2:w322, 3:w327) -> (0:w323:i32)  [unwired: 1 out]
                n200 = property on="Test Ring" class="Ring (strict)"("Value"=w323, "Strings []"=w322) -> ()  [unwired: 2 in, 2 out]
                n201 = property on="Test Ring" class="Ring (strict)"("Visible"=TRUE) -> ()  [unwired: 2 in, 2 out]
                n202 = property on="Test Slider" class="Slide (strict)"("Visible"=FALSE) -> ()  [unwired: 2 in, 2 out]
              }
              frame Default {
                n203 = property on="Test Ring" class="Ring (strict)"("Visible"=FALSE) -> ()  [unwired: 2 in, 2 out]
                n204 = property on="Test Slider" class="Slide (strict)"("Visible"=FALSE) -> ()  [unwired: 2 in, 2 out]
              }
              frame "Brightness  **", "Color Level  **", "Compression  **", "FPS  **", "Sharpness  **" {
                n205 = call <vilib>:"NT Read Number.vi"("Name"=w334) -> ("Numeric"=w333:dbl)  [unwired: 9 in, 1 out]
                n206 = local write "Test Slider"(w333) -> ()
                n207 = property on="Test Slider" class="Slide (strict)"("Visible"=TRUE, "Scale.Maximum"=100.0 ("Scale.Range:Maximum")) -> ()  [unwired: 2 in, 2 out]
                n208 = property on="Test Ring" class="Ring (strict)"("Visible"=FALSE) -> ()  [unwired: 2 in, 2 out]
              }
            }
          }
        }
        n209 = property on="Progress" class="Clust (strict)"("Visible"=FALSE) -> ()  [unwired: 2 in, 2 out]
      }
      event "Test Name": Mouse Enter {
        # "Populate the ring with the list of tests"
        n210 = event-data() -> ()  [unwired: 1 in, 1 out]
        n211 = call <vilib>:"NT Read String Array.vi"("Name"="/TestMode/TestList") -> ("String Array"=w342:string[])  [unwired: 9 in, 1 out]
        n212 = Build Array (concatenate)("Select the test to run...", w342) -> (w341:string[])
        n213 = property on="Test Name" class="Ring (strict)"("Strings []"=w341) -> ()  [unwired: 2 in, 2 out]
      }
      event "Test Name": Value Change {
        w344 = FALSE ("Visible")
        # "Tell the robot the test name to run"
        n214 = event-data() -> ("NewVal"=w348:u16)  [unwired: 1 in]
        n215 = property on="Test Name" class="Ring (strict)"() -> ("Strings []"=w349:string[])  [unwired: 2 in, 2 out]
        n216 = local write "Progress"(T6 {"Test Progress"=0, "Test Progress Text"=""} ("Progress")) -> ()
        n217 = Index Array(array=w349, index=w348) -> (element=w347:string)
        n218 = call <vilib>:"NT Write String.vi"("String"=w347, "Name"="/TestMode/TestName") -> ()  [unwired: 9 in, 1 out]
        n219 = property on="Progress" class="Clust (strict)"("Visible"=TRUE) -> ()  [unwired: 2 in, 2 out]
        n220 = property on="Motor" class="Clust (strict)"("Visible"=w344) -> ()  [unwired: 2 in, 2 out]
        n221 = property on="Test Slider" class="Slide (strict)"("Visible"=w344) -> ()  [unwired: 2 in, 2 out]
        n222 = property on="On/Off" class="Bool (strict)"("Visible"=w344) -> ()  [unwired: 2 in, 2 out]
        n223 = property on="Rev/Fwd" class="Clust (strict)"("Visible"=w344) -> ()  [unwired: 2 in, 2 out]
        n224 = property on="Test Ring" class="Ring (strict)"("Visible"=w344) -> ()  [unwired: 2 in, 2 out]
      }
      event "Select Auto": Mouse Enter {
        # "Populate the combo box with the list of autonomous options"
        n225 = event-data() -> ()  [unwired: 1 in, 1 out]
        n226 = call <vilib>:"NT Read String Array.vi"("Name"="Auto List") -> ("String Array"=w351:string[])  [unwired: 9 in, 1 out]
        n227 = property on="Select Auto" class="CmbBox"("Strings[]"=w351) -> ()  [unwired: 2 in, 2 out]
      }
      event "Select Auto": Value Change {
        # "User modified the Auto Selection. Write to NT variable so robot knows."
        n228 = event-data() -> ("NewVal"=w354:string)  [unwired: 1 in]
        n229 = call <vilib>:"NT Write String.vi"("String"=w354, "Name"="Auto Selector") -> ()  [unwired: 9 in, 1 out]
      }
      event "Command Selection": Value Change {
        # "Get the params and show in table"
        n230 = event-data() -> ("NewVal"=w360:i32)  [unwired: 1 in]
        n231 = property on="Command Selection" class="MCListbox (strict)"() -> ("ItemNames"=w358:string[][])  [unwired: 2 in, 2 out]
        n232 = call <vilib>:"WPI_DashboardUpdate Command Params.vi"("NewVal"=w360, "Commands"=w358, "Param Tbl"=w359) -> ()  [unwired: 8 in, 1 out]
      }
      event "Execute Command": Value Change {
        # "Started one, Unique ID holds\nresponse"
        n233 = event-data() -> ()  [unwired: 1 in, 1 out]
        n234 = property on="Command Selection" class="MCListbox (strict)"() -> ("ItemNames"=w371:string[][])  [unwired: 2 in, 2 out]
        n235 = Index Array(array=w371, index (row)="Command Selection", index (col)=0) -> (element=w369:string)
        n236 = call <vilib>:"Invoke Commands.vi"("Command Params"="Command Params", "Function Name"=w369) -> ("Params"=w365:u8, "Started"=w364:bool)  [unwired: 7 in, 1 out]
        n237 = Array Subset(array="Command Params", length (row)=w365) -> (w366:string[][])  [unwired: 3 in]
        n238 = Select(t="Executing" ("Cmd Status"), s=w364, f="" ("Cmd Status")) -> (s? t:f=→"Cmd Status":string)
      }
      event "Command Selection": Double Click {
        n239 = event-data() -> ("Row"=w379:i32)  [unwired: 1 in]
        n240 = property on="Command Selection" class="MCListbox (strict)"() -> ("ItemNames"=w382:string[][])  [unwired: 2 in, 2 out]
        n241 = local read "Command Params"() -> (w378:string[][])
        n242 = Index Array(array=w382, index (row)=w379, index (col)=0) -> (element=w380:string)
        n243 = call <vilib>:"Invoke Commands.vi"("Command Params"=w378, "Function Name"=w380) -> ("Params"=w377:u8, "Started"=w372:bool)  [unwired: 7 in, 1 out]
        n244 = Array Subset(array=w378, length (row)=w377) -> (w376:string[][])  [unwired: 3 in]
        n245 = Select(t="Executing" ("Cmd Status"), s=w372, f="" ("Cmd Status")) -> (s? t:f=w373:string)
        n246 = local write "Cmd Status"(w373) -> ()
      }
      event "CheckList": Double Click {
        # "Shift clears all"
        # "Update symbols on the listbox"
        n247 = event-data() -> ("PlatMods.Shift"=w384:bool, "Row"=w386:i32)  [unwired: 1 in]
        n248 = case shown="True" w384 {
          tunnel: w386 -> [w390 _]
          tunnel: 1 -> [w389 _]
          frame False {
            n249 = property on="CheckList" class="LstBox (strict)"() -> ("Item Symbols"=w388:i32[])  [unwired: 2 in, 2 out]
            n250 = Replace Array Subset(array=w388, new element=w389, index=w390) -> (w387:i32[])
            n251 = property on="CheckList" class="LstBox (strict)"("Item Symbols"=w387) -> ()  [unwired: 2 in, 2 out]
          }
          frame True {
            w391 = 0 ("Top Row")
            n252 = property on="CheckList" class="LstBox (strict)"() -> ("Number of Rows"=w393:u32)  [unwired: 2 in, 2 out]
            n253 = Initialize Array(0, w393) -> (w392:i32[])
            n254 = property on="CheckList" class="LstBox (strict)"("Top Row"=w391, "Value"=w391, "Item Symbols"=w392) -> ()  [unwired: 2 in, 2 out]
          }
        }
      }
      event "CheckList": Key Down {
        # "Update symbols on the listbox\nLeft and right keys check and uncheck"
        n255 = event-data() -> ("VKey"=w397:T19)  [unwired: 1 in]
        n256 = case shown="\"Left\", \"Right\"" w397 {
          selector: w397 -> [w402 _]
          tunnel: eventvkey."Left" ("VKey") -> [w400 _]
          frame "Left", "Right" {
            n257 = Equal?(x=w400, y=w402) -> (x = y?=w401:bool)
            n258 = Select(t=0, s=w401, f=1) -> (s? t:f=w403:i32)
            n259 = property on="CheckList" class="LstBox (strict)"() -> ("Item Symbols"=w406:i32[])  [unwired: 2 in, 2 out]
            n260 = Replace Array Subset(array=w406, new element=w403, index="CheckList") -> (w405:i32[])
            n261 = property on="CheckList" class="LstBox (strict)"("Item Symbols"=w405) -> ()  [unwired: 2 in, 2 out]
          }
          frame Default {
          }
        }
      }
      event "Motor.Enable": Value Change {
        # "When the test mode otor enable helper is set, update that\ntree row item's value"
        n262 = event-data() -> ("NewVal"=w412:bool)  [unwired: 1 in]
        n263 = Unbundle("Motor") -> ("Value"=w411:dbl)  [unwired: 1 out]
        n264 = Select(t=w411, s=w412, f=0.0) -> (s? t:f=w409:dbl)
        n265 = call <vilib>:"NT Write Number.vi"("Numeric"=w409, "Name"=w408) -> ()  [unwired: 9 in, 1 out]
      }
      event "Test Slider": Value Change {
        # "When the test mode slider helper is set, update that\ntree row item's value"
        n266 = event-data() -> ("NewVal"=w415:dbl)  [unwired: 1 in]
        n267 = call <vilib>:"NT Write Number.vi"("Numeric"=w415, "Name"=w416) -> ()  [unwired: 9 in, 1 out]
      }
      event "On/Off": Value Change {
        # "When the test mode on/off helper value is set, update that\ntree row item's value"
        n268 = event-data() -> ("NewVal"=w420:bool)  [unwired: 1 in]
        n269 = Boolean To (0,1)(Boolean=w420) -> (0, 1=w419:i16)
        n270 = call <vilib>:"NT Write Number.vi"("Numeric"=w419, "Name"=w418) -> ()  [unwired: 9 in, 1 out]
      }
      event "Rev/Fwd": Value Change {
        # "When the test mode helper value for relays is set, update that\ntree row item's value"
        n271 = event-data() -> ("NewVal.Forward"=w428:bool, "NewVal.Reverse"=w427:bool)  [unwired: 1 in]
        n272 = Boolean To (0,1)(Boolean=w428) -> (0, 1=w424:i16)
        n273 = Boolean To (0,1)(Boolean=w427) -> (0, 1=w426:i16)
        n274 = Negate(x=w426) -> (-x=w425:i16)
        n275 = Add(x=w424, y=w425) -> (x+y=w423:i16)
        n276 = call <vilib>:"NT Write Number.vi"("Numeric"=w423, "Name"=w422) -> ()  [unwired: 9 in, 1 out]
      }
      event "Test Ring": Value Change {
        # "When a test mode helper value is selected from the ring,\nset the tree item's variable to the string value"
        n277 = event-data() -> ("NewVal"=w432:u16)  [unwired: 1 in]
        n278 = property on="Test Ring" class="Ring (strict)"() -> ("Strings []"=w433:string[])  [unwired: 2 in, 2 out]
        n279 = Index Array(array=w433, index=w432) -> (element=w431:string)
        n280 = call <vilib>:"NT Write String.vi"("String"=w431, "Name"=w430) -> ()  [unwired: 9 in, 1 out]
      }
      event "Rec Mode": Value Change {
        # "Update globals for recording mode and path to read log from.\nClear when logging and let NetworkTables set path for vision to\nuse."
        n281 = event-data() -> ("NewVal"=w444:enum32{"Stop", "Record", "Playback"})  [unwired: 1 in]
        n282 = global write "WPI_DashboardLogging Global.vi" "Logging Filename"(path "") -> ()
        n283 = global write "WPI_DashboardLogging Global.vi" "Recording"(w444) -> ()
        n284 = case shown="\"Playback\"" w444 {
          tunnel: w443 -> [_ w446 w455]
          tunnel: [_ _ w454] -> w441
          tunnel: [_ _ w453] -> _
          tunnel: w439 -> [_ _ w451]
          tunnel: cluster{i32, i32} {-250, 170} -> [_ _ w450]
          tunnel: [_ _ T20 {"Image Size"=TRUE, "Image Type"=TRUE, "Pixel Value"=TRUE, "ROI Information"=TRUE, "Zoom Factor"=FALSE} ("Image Information Shown:All Elements")] -> w437
          tunnel: [_ _ TRUE ("Zoom Factor")] -> w436
          tunnel: w435 -> [_ _ w447]
          frame Default {
          }
          frame "Stop", "Record" {
            # "Place Window too"
            n285 = invoke class="VI" method="FP.Close"(reference=w446) -> (reference out=w445:refnum<vi>)  [unwired: 2 in, 2 out]
            n286 = invoke class="VI" method="Abort VI"(reference=w445) -> ()  [unwired: 2 in, 3 out]
          }
          frame "Playback" {
            n287 = call "Open Playback Panel.vi"("Offset"=w450, "DB VI Ref"=w451, "Playback in"=w455) -> ("Playback out"=w452:refnum<vi>)  [unwired: 8 in]
            n288 = register-events(w452, w447) -> (reference out=w454:refnum<event-registration>, error out=w453:errorcluster)  [unwired: 2 in]
          }
        }
        n289 = property on="Camera Image" class="ImageControl"("Image Information Shown"=w437, "Image Information Visible"=w436) -> ()  [unwired: 2 in, 2 out]
        n290 = call <vilib>:"WPI_DashboardNT Log FieldName Cache.vi"("Operation"=enum16{"Lookup/Add", "Index", "Clear"}."Clear") -> ()  [unwired: 8 in, 3 out]
      }
      event Panel Close {
        w457 = enum32{"Stop", "Record", "Playback"}."Stop" ("Rec Mode")
        # "Playback window has been closed, abort"
        n291 = event-data() -> ()  [unwired: 1 in, 4 out]
        n292 = local write "Rec Mode"(w457) -> ()
        n293 = global write "WPI_DashboardLogging Global.vi" "Recording"(w457) -> ()
      }
      event Panel Close {
        # "Abort playback window and ourself"
        n294 = event-data() -> ()  [unwired: 1 in, 4 out]
        n295 = invoke class="VI" method="FP.Close"(reference=w461) -> (reference out=w460:refnum<vi>)  [unwired: 2 in, 2 out]
        n296 = invoke class="VI" method="Abort VI"(reference=w460) -> (error out=w459:errorcluster)  [unwired: 2 in, 2 out]
        n297 = invoke class="VI" method="Abort VI"(error in=w459) -> ()  [unwired: 2 in, 3 out]
      }
      event User Event {
        n298 = event-data() -> ("IDs"=w468:cluster{"RPC field ID":u16, "Unique ID":u16}, "String"=w467:string)  [unwired: 1 in]
        n299 = Bundle("IDs"=w468, "String"=w467) -> (w466:T8)  [unwired: 1 in]
        n300 = call <vilib>:"Retrieve RPC Response.vi"("RPC Response"=w466) -> ("Output"=w464:string[][])  [unwired: 10 in]
        n301 = Build Array (concatenate)(w462, w464) -> (w463:string[][])
        n302 = local write "Command Params"(w463) -> ()
        n303 = local write "Cmd Status"("" ("Cmd Status")) -> ()
      }
      event "Tree": Double Click {
        n304 = event-data() -> ("PlatMods"=w472:T23, "Tag"=w471:string)  [unwired: 1 in]
        n305 = Unbundle(w472) -> ("Shift"=w470:bool)  [unwired: 4 out]
        n306 = Not(x=w470) -> (.not. x?=w469:bool)
        n307 = call <vilib>:"NT Update Persistence.vi"("Persistence"=w469, "Name"=w471) -> ()  [unwired: 9 in, 1 out]
      }
    }
  }
  n308 = while {
    tunnel: w64 -> [w475]
    i -> [w478]
    stop <- FALSE stop-if-true
    n309 = Wait (ms)(milliseconds to wait=u32 100) -> ()  [unwired: 1 out]
    n310 = case shown="\"Playback\"" "Rec Mode" {
      tunnel: w478 -> [_ _ w493]
      tunnel: [u32 2829099 ("Base Color") u32 11141120 ("Target Color") w482] -> w474
      frame "Stop", Default {
        # "Reset the color, extra updates don't cost much"
      }
      frame "Record" {
      }
      frame "Playback" {
        # "Playback"
        n311 = Quotient & Remainder(x=w493, y=u32 50 ("milliseconds to wait")) -> (x-y*floor(x/y)=w489:u32)  [unwired: 1 out]
        n312 = Divide(x=w489, y=u32 50 ("milliseconds to wait")) -> (x/y=w486:dbl)
        n313 = Multiply(x=6.283185307179586, y=w486) -> (x*y=w491:dbl)
        n314 = Sine(x=w491) -> (sin(x)=w490:dbl)
        n315 = Absolute Value(x=w490) -> (abs(x)=w483:dbl)
        n316 = call "Interpolate RGB Color.vi"("Proportion"=w483, "Target Color"=u32 30976, "Base Color"=u32 2829099) -> ("Result Color"=w482:u32)  [unwired: 8 in]
      }
    }
    n317 = property class="Pane"(reference=w475, "PaneColor"=w474) -> ()  [unwired: 1 in, 2 out]
  }
  n318 = local write "Dashboard Tab"(T2."Drive" ("Dashboard Tab")) -> ()
  n319 = property on="On/Off" class="Bool (strict)"("Visible"=w33) -> ()  [unwired: 2 in, 2 out]
  n320 = property on="Motor" class="Clust (strict)"("Visible"=w33) -> ()  [unwired: 2 in, 2 out]
  n321 = property on="Progress" class="Clust (strict)"("Visible"=w33) -> ()  [unwired: 2 in, 2 out]
  n322 = property on="Test Ring" class="Ring (strict)"("Visible"=w33) -> ()  [unwired: 2 in, 2 out]
  n323 = property on="Rev/Fwd" class="Clust (strict)"("Visible"=w33) -> ()  [unwired: 2 in, 2 out]
  n324 = while {
    tunnel: u16 1741 ("timeout ms (25000)") -> [w495]
    stop <- FALSE stop-if-true
    n325 = TCP Create Listener(10:w495) -> (0:w494:errorcluster, 3:w496:refnum<k5>)  [unwired: 4 in, 1 out]
    n326 = case shown="No Error" w494 {
      selector: w494 -> [w498 _]
      tunnel: w496 -> [w499 _]
      frame No Error {
        n327 = while {
          tunnel: w499 -> [w502]
          tunnel: w498 -> [w501]
          stop <- FALSE stop-if-true
          n328 = TCP Wait On Listener(8:w501, 11:w502) -> (0:w503:errorcluster, 4:w504:refnum<k5>)  [unwired: 2 in, 3 out]
          n329 = local write "TCP"(w504) -> ()
          n330 = case shown="No Error" w503 {
            frame No Error {
            }
            frame Error {
              n331 = Wait (ms)(milliseconds to wait=u32 1000) -> ()  [unwired: 1 out]
            }
          }
        }
      }
      frame Error {
        n332 = Wait (ms)(milliseconds to wait=u32 1000) -> ()  [unwired: 1 out]
      }
    }
  }
  n333 = local write "Command Selection"(u16 0 ("milliseconds to wait")) -> ()
  n334 = local write "Command Params"(string[][] [] ("Command Params")) -> ()
  n335 = global write "WPI_DashboardLogging Global.vi" "Recording"(w58) -> ()
  n336 = local write "Rec Mode"(w58) -> ()
  n337 = call <vilib>:"NT Write String.vi"("String"="Select Auto", "Name"="Auto Selector") -> ()  [unwired: 9 in, 1 out]
